vi "daqio_Connection_FGV.vi"(6 "Connection Status in":T1=enum."Connected", 8 "error in":errorcluster, 9 "Buffered Data exists":bool, 10 "Enum":T2=enum."Set Type", 11 "daq.io type in":T3={"daq.io ref"=refnum, "daq.io API Base"="http://dashboard.daq.io/api/v1", "Device Key"="DESKTOP_7UDDDR9_LOCALDOMAIN_TYPE", "Account ID"="DESKTOP_7UDDDR9_LOCALDOMAIN", "online"=TRUE, "SSL"=TRUE}) -> (0 "error out":errorcluster, 1 "Buffered Data exists?":bool, 3 "daq.io type out":T3={"daq.io ref"=refnum, "daq.io API Base"="", "Device Key"="", "Account ID"="", "online"=TRUE, "SSL"=FALSE}, 4 "Connection Status out":T1)   [LabVIEW 2013, in "daqio minimal.lvlib"]
doc: "This VI is a functional global variable that stores all relevant daq.io connection data.\n\nIt stores the daq.io connection data, such as the current Device Key, the Account ID, whether or not the device is online.\n\nIt also contains the connection status information (whether it was re-connected recently)\n\nAlso, it is used to exchange data whether buffered data exists and needs to be uploaded once the device reconnects."
uses:
  daqio minimal.lvlib
  _typedefs/daqio-Type.ctl
  <vilib>/httpClient/ClientHandle.ctl
  _typedefs/connection_FGV_commands.ctl
  _typedefs/daqio-reconnect-status.ctl
  <vilib>/httpClient/LabVIEWHTTPClient.lvlib
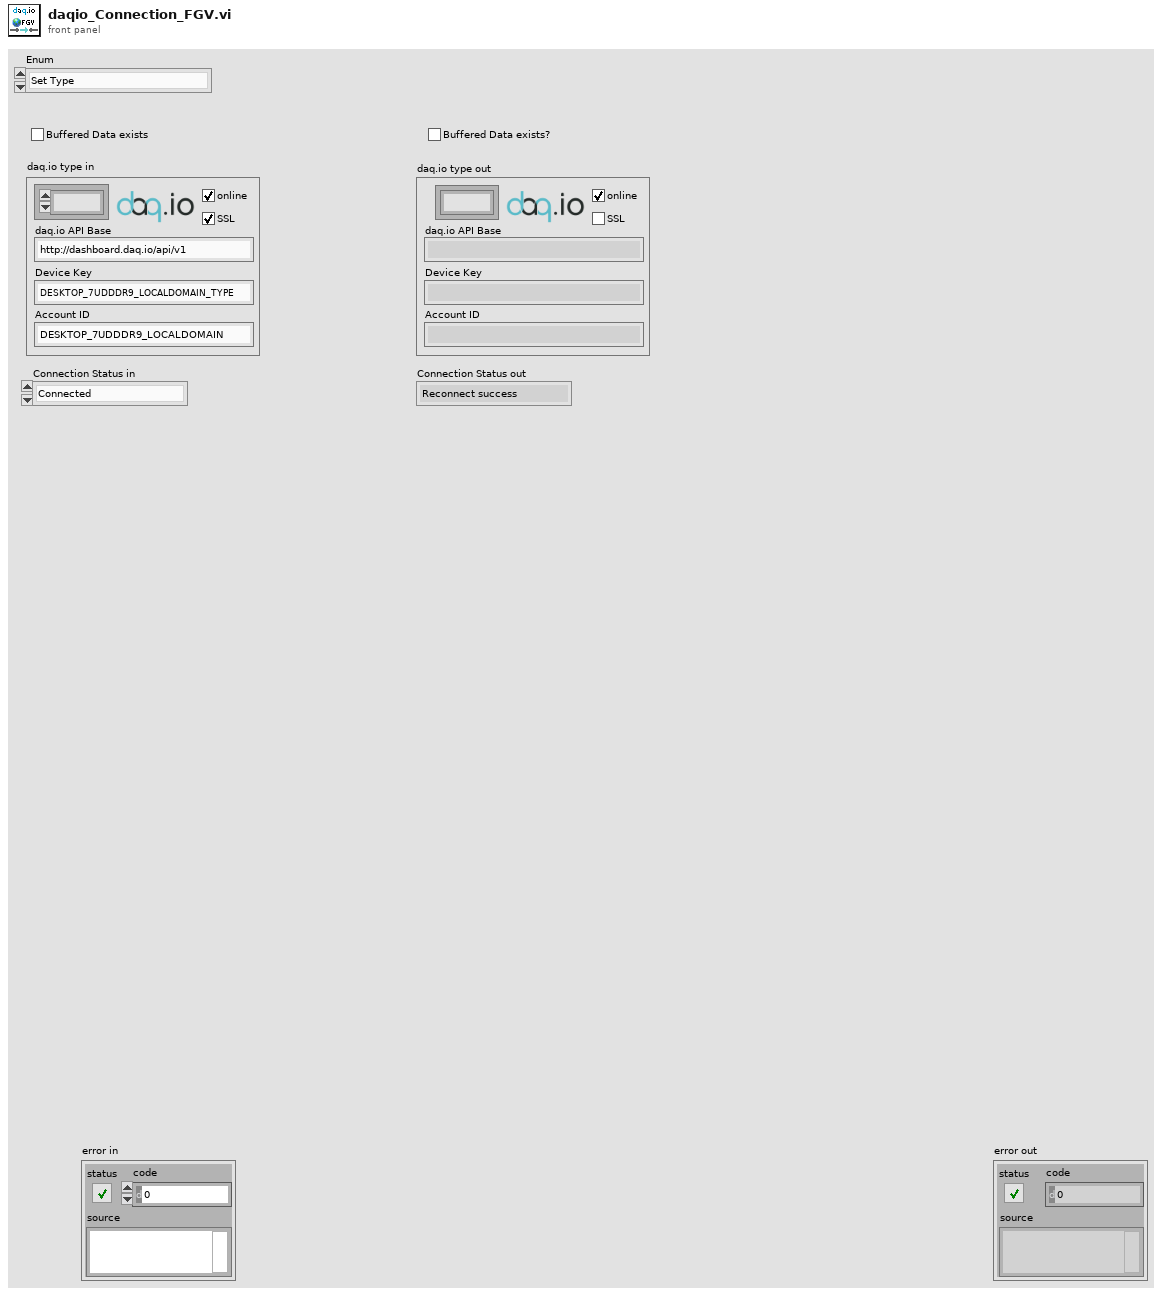
[diagram p1: front panel]
types:
  T1 = typedef "daqio minimal.lvlib/daqio-reconnect-status.ctl" = enum16{"Reconnect success", "Reconnect failed", "Connected", "Offline"}
  T2 = typedef "daqio minimal.lvlib/connection_FGV_commands.ctl" = enum16{"Set Conn Stat", "Save Type", "Get Type from File", "Set Type", "Set Buffer", "Get"}
  T3 = typedef "daqio minimal.lvlib/daqio-Type.ctl" = cluster{"daq.io ref":T4, "daq.io API Base":string, "Device Key":string, "Account ID":string, "online":bool, "SSL":bool}
  T4 = typedef "LabVIEWHTTPClient.lvlib/ClientHandle.ctl" = refnum<k1>
  T5 = enum16{"open", "replace", "create", "open or create", "replace or create", "replace or create with confirmation"}
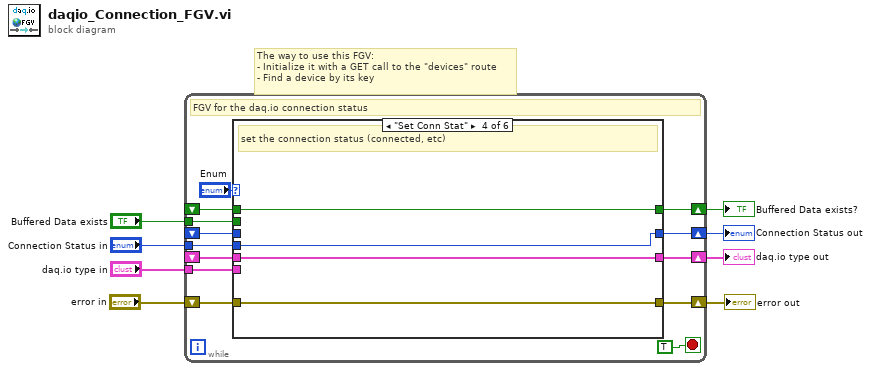
[diagram p0: block diagram]
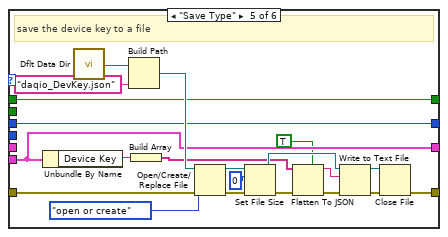
[diagram p5: hidden frame]
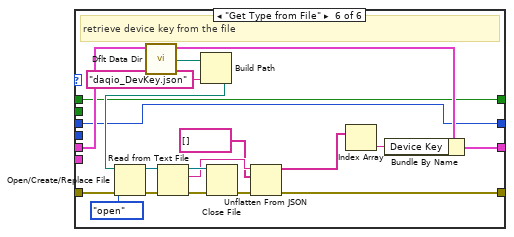
[diagram p6: hidden frame]
diagram:
  # "The way to use this FGV: \n- Initialize it with a GET call to the \"devices\" route\n- Find a device by its key"
  n1 = while {
    shift-right: [w20] -> w5
    shift-left: _ -> [w19]
    shift-right: [w10] -> w7
    shift-left: "error in" -> [w9]
    tunnel: "daq.io type in" -> [w18]
    shift-right: [w17] -> w3
    shift-left: _ -> [w16]
    tunnel: "Buffered Data exists" -> [w15]
    tunnel: "Connection Status in" -> [w12]
    shift-right: [w13] -> w1
    shift-left: _ -> [w11]
    stop <- TRUE stop-if-true
    # "FGV for the daq.io connection status"
    n2 = case shown="\"Set Conn Stat\"" "Enum" {
      tunnel: [w25 w29 w32 w36 w43 w65] -> w20
      tunnel: w19 -> [_ w29 w32 w36 _ w66]
      tunnel: w18 -> [w25 _ _ _ w43 _]
      tunnel: [w24 w28 w33 w35 w41 w63] -> w17
      tunnel: w16 -> [w24 w28 _ w35 w41 w63]
      tunnel: w15 -> [_ _ w33 _ _ _]
      tunnel: [w23 w27 w31 w37 w42 w62] -> w13
      tunnel: w12 -> [_ _ _ w37 _ _]
      tunnel: w11 -> [w23 w27 w31 _ w42 w62]
      tunnel: [w22 w26 w30 w34 w44 w64] -> w10
      tunnel: w9 -> [w22 w26 w30 w34 w45 w73]
      frame "Set Type" {
        # "set the daq.io connection info"
      }
      frame "Get", Default {
        # "get all stored status information"
      }
      frame "Set Buffer" {
        # "switch flag on that buffered data exists"
      }
      frame "Set Conn Stat" {
        # "set the connection status (connected, etc)"
      }
      frame "Save Type" {
        # "save the device key to a file"
        n3 = Unbundle By Name(w43) -> ("Device Key"=w39:string)
        n4 = call <vilib>:"Dflt Data Dir.vi"() -> ("App:Default Data Directory"=w57:path)
        n5 = Build Path(base path=w57, name or relative path="daqio_DevKey.json") -> (appended path=w55:path)
        n6 = Build Array(w39) -> (w38:string[])
        n7 = Open/Create/Replace File(file path (use dialog)=w55, error in=w45, operation (0:open)=T5."open or create") -> (refnum out=w52:refnum<file>, error out=w54:errorcluster)  [unwired: 3 in, 1 out]
        n8 = Set File Size(4:w54, 6:i64 0 ("size (in bytes)"), 7:w52) -> (0:w51:errorcluster, 3:w49:refnum<file>)
        n9 = Flatten To JSON(enable LabVIEW extensions? (T)=TRUE, anything=w38, error in (no error)=w51) -> (JSON string=w50:string, 11:w48:errorcluster)
        n10 = Write to Text File(file (use dialog)=w49, text=w50, error in=w48) -> (refnum out=w46:refnum<file>, error out=w47:errorcluster)  [unwired: 1 in, 1 out]
        n11 = Close File(refnum=w46, error in=w47) -> (error out=w44:errorcluster)  [unwired: 1 out]
      }
      frame "Get Type from File" {
        # "retrieve device key from the file"
        n12 = call <vilib>:"Dflt Data Dir.vi"() -> ("App:Default Data Directory"=w76:path)
        n13 = Build Path(base path=w76, name or relative path="daqio_DevKey.json") -> (appended path=w74:path)
        n14 = Open/Create/Replace File(file path (use dialog)=w74, error in=w73, operation (0:open)=T5."open") -> (refnum out=w69:refnum<file>, error out=w72:errorcluster)  [unwired: 3 in, 1 out]
        n15 = Read from Text File(file (use dialog)=w69, error in=w72) -> (refnum out=w70:refnum<file>, text=w67:string, error out=w71:errorcluster)  [unwired: 2 in, 1 out]
        n16 = Close File(refnum=w70, error in=w71) -> (error out=w68:errorcluster)  [unwired: 1 out]
        n17 = Unflatten From JSON(JSON string=w67, type and defaults=string[] [], error in (no error)=w68) -> (value=w60:string[], error out=w64:errorcluster)  [unwired: 4 in]
        n18 = Index Array(array=w60) -> (element=w59:string)  [unwired: 1 in]
        n19 = Bundle By Name(cluster=w66, "Device Key"=w59) -> (w65:T3)
      }
    }
  }
  "error out" <- w7
  "daq.io type out" <- w5
  "Buffered Data exists?" <- w3
  "Connection Status out" <- w1
